vi "JSON to LVObject - Error Input - Returns Object Type.vi"() -> ()   [LabVIEW 2017, in "JSON Serializable Serializer Tests.lvlib"]
uses:
  JSON Serializable Serializer Tests.lvlib
  Mock JSON Serializable/Mock JSON Serializable.lvclass
  JSON Serializable Serializer/JSON Serializable Serializer.lvclass
  <vilib>/Utility/error.llb/Error Cluster From Error Code.vi
  <vilib>/addons/_JKI Toolkits/Caraya/classes/Assert/Assert Equal Value_Variant.vi
  <vilib>/ErrorRing/Error Ring.xnode
  <vilib>/addons/_JKI Toolkits/Caraya/classes/Test/Test.lvclass
  <vilib>/addons/_JKI Toolkits/Caraya/classes/Assert/Assert.lvclass
panel:
  out "error out":errorcluster
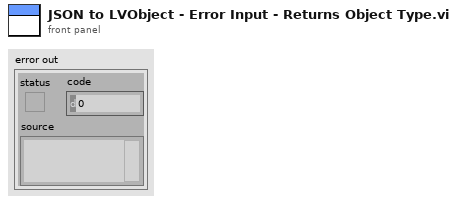
[diagram p1: front panel]
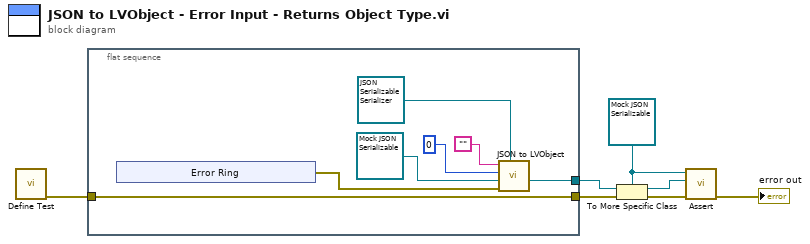
[diagram p0: block diagram]
diagram:
  w1 = refnum<class "Mock JSON Serializable.lvclass"> refnum ("JSON Serializer Tests.lvlib:Mock JSON Serializable.lvclass")
  n1 = call <vilib>:"Define Test.vi"() -> ("error out"=w6:errorcluster)  [unwired: 11 in]
  n2 = flat-sequence {
    tunnel: [w13] -> w7
    tunnel: w6 -> [w13]
    tunnel: [w8] -> w3
    frame #0 {
      n3 = xnode "Error Ring"() -> ("error out"=w14:errorcluster)
      n4 = call-dynamic "JSON to LVObject.vi"("JSON Serializer in"=refnum<class "JSON Serializable Serializer.lvclass"> refnum ("JSON Serializer.lvclass"), "error in (no error)"=w14, "Object Type"=refnum<class "Mock JSON Serializable.lvclass"> refnum ("Type"), "Offset"=0, "JSON"="") -> ("Object"=w8:refnum<class>)  [unwired: 5 in, 1 out]
    }
  }
  n5 = To More Specific Class(target class=w1, reference=w3, error in=w7) -> (specific class reference=w2:refnum<class "Mock JSON Serializable.lvclass">, error out=w4:errorcluster)
  n6 = call-poly <vilib>:"Assert.vi"("error in (no error)"=w4, "Y"=w2, "X"=w1) -> ("error out"=→"error out":errorcluster)  [unwired: 8 in]
